vi "BRig_dataRT_stats__TpB_target.vi"() -> (2 "output_TpB_target":i32)   [LabVIEW 2014]
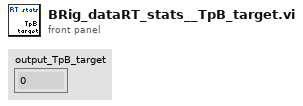
[diagram p1: front panel]
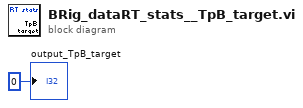
[diagram p0: block diagram]
diagram:
  "output_TpB_target" <- 0 ("output_iBlock")
